vi "Query System State.vi"(8 "error in (no error)":errorcluster, 10 "Channel (1:CH1)":u16(ring)=1 items=["CH1"=1, "CH2"=2], 11 "VISA resource name":refnum<visa-resource-name>) -> (0 "error out":errorcluster, 1 "Output Mode":string, 2 "Operation Mode":string, 3 "VISA resource name out":refnum<visa-resource-name>, 5 "Waveform Display":bool, 6 "Timer":bool, 7 "Output Status":bool)   [LabVIEW 2015, in "Siglent SPD3000 Series.lvlib"]
doc: "Returns status for a desired channel."
uses:
  <instrlib>/Siglent SPD3000 Series/Siglent SPD3000 Series.lvlib
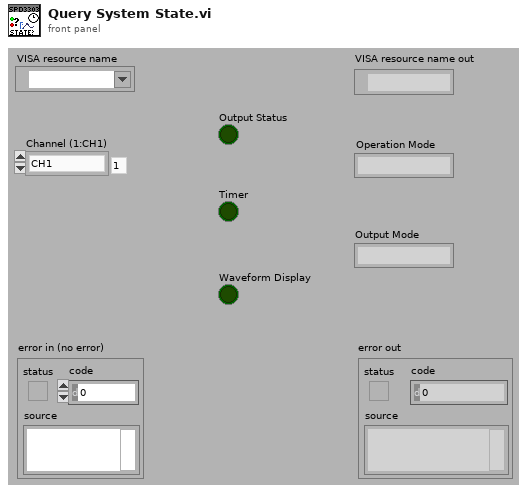
[diagram p1: front panel]
types:
  T1 = cluster{"Boolean array[0]":bool, "Boolean array[1]":bool, "Boolean array[2]":bool, "Boolean array[3]":bool, "Boolean array[4]":bool, "Boolean array[5]":bool, "Boolean array[6]":bool, "Boolean array[7]":bool, "Boolean array[8]":bool, "Boolean array[9]":bool}
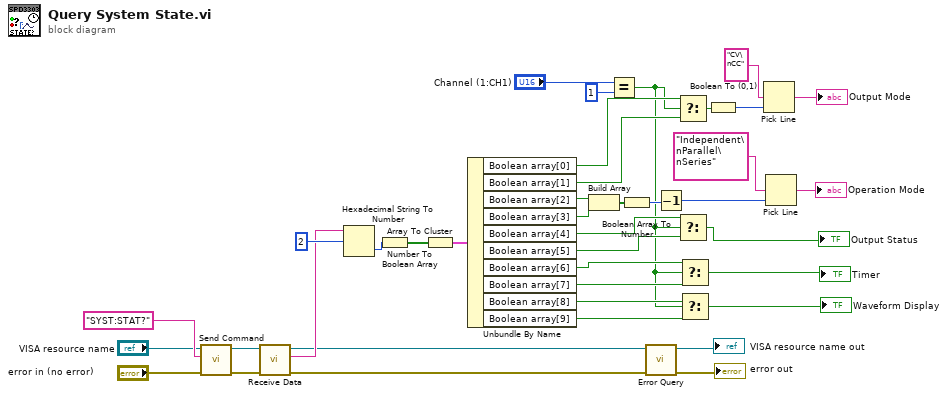
[diagram p0: block diagram]
diagram:
  n1 = call <instrlib>:"Send Command.vi"("error in (no error)"="error in (no error)", "Write Buffer (\"\")"="SYST:STAT?" ("Command"), "VISA resource name"="VISA resource name") -> ("error out"=w37:errorcluster, "VISA resource name out"=w36:refnum<visa-resource-name>)  [unwired: 7 in]
  n2 = call <instrlib>:"Receive Data.vi"("error in (no error)"=w37, "VISA resource name"=w36) -> ("error out"=w6:errorcluster, "Read Buffer"=w27:string, "VISA resource name out"=w7:refnum<visa-resource-name>)  [unwired: 6 in, 1 out]
  n3 = Hexadecimal String To Number(string=w27, offset=2 ("偏移量")) -> (number=w29:u32)  [unwired: 1 in, 1 out]
  n4 = Number To Boolean Array(number=w29) -> (Boolean array=w30:bool[])
  n5 = Array To Cluster(array=w30) -> (cluster=w28:T1)
  n6 = Unbundle By Name(w28) -> ("Boolean array[0]"=w23:bool, "Boolean array[1]"=w24:bool, "Boolean array[2]"=w34:bool, "Boolean array[3]"=w33:bool, "Boolean array[4]"=w22:bool, "Boolean array[5]"=w21:bool, "Boolean array[6]"=w19:bool, "Boolean array[7]"=w18:bool, "Boolean array[8]"=w16:bool, "Boolean array[9]"=w15:bool)
  n7 = Build Array(w34, w33) -> (w32:bool[])
  n8 = Equal?(x="Channel (1:CH1)", y=u16 1) -> (x = y?=w14:bool)
  n9 = Boolean Array To Number(Boolean array=w32) -> (number=w31:u32)
  n10 = call <instrlib>:"Error Query.vi"("error in (no error)"=w6, "VISA resource name"=w7) -> ("error out"=→"error out":errorcluster, "VISA resource name out"=→"VISA resource name out":refnum<visa-resource-name>)  [unwired: 6 in, 2 out]
  n11 = Decrement(x=w31) -> (x-1=w26:u32)
  n12 = Select(t=w23, s=w14, f=w24) -> (s? t:f=w11:bool)
  n13 = Select(t=w22, s=w14, f=w21) -> (s? t:f=→"Output Status":bool)
  n14 = Select(t=w19, s=w14, f=w18) -> (s? t:f=→"Timer":bool)
  n15 = Select(t=w16, s=w14, f=w15) -> (s? t:f=→"Waveform Display":bool)
  n16 = Boolean To (0,1)(Boolean=w11) -> (0, 1=w9:i16)
  n17 = Pick Line(multi-line string="CV\nCC" ("多行字符串"), line index=w9) -> (output string=→"Output Mode":string)  [unwired: 1 in]
  n18 = Pick Line(multi-line string="Independent\nParallel\nSeries" ("字符串(\"\")"), line index=w26) -> (output string=→"Operation Mode":string)  [unwired: 1 in]
